vi "process_display.vi"(6 "error in (no error)":errorcluster) -> (0 "error out":errorcluster)   [LabVIEW 2010]
uses:
  typedefs/control_display_enum.ctl
  typedefs/data_array.ctl
panel:
  out "Waveform Chart":waveform(dbl)[](graph)
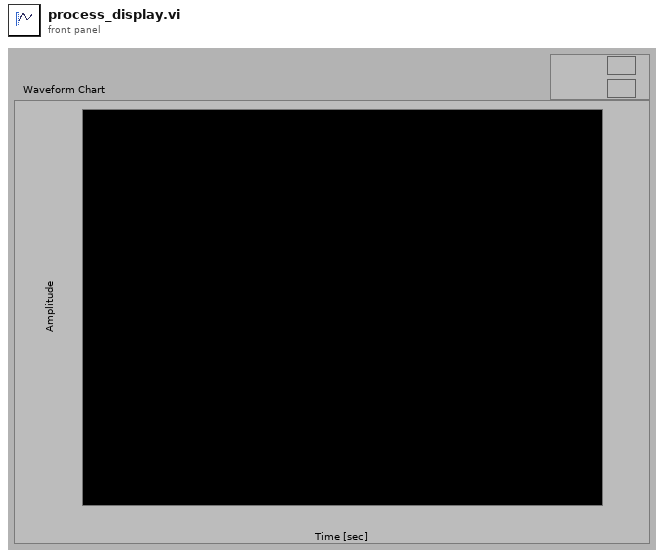
[diagram p1: front panel]
types:
  T1 = typedef "data_array.ctl" = waveform(dbl)[]
  T2 = typedef "control_display_enum.ctl" = enum16{"Init", "Display", "Quit"}
  T3 = cluster{"Control display enum":T2, "variant":variant}
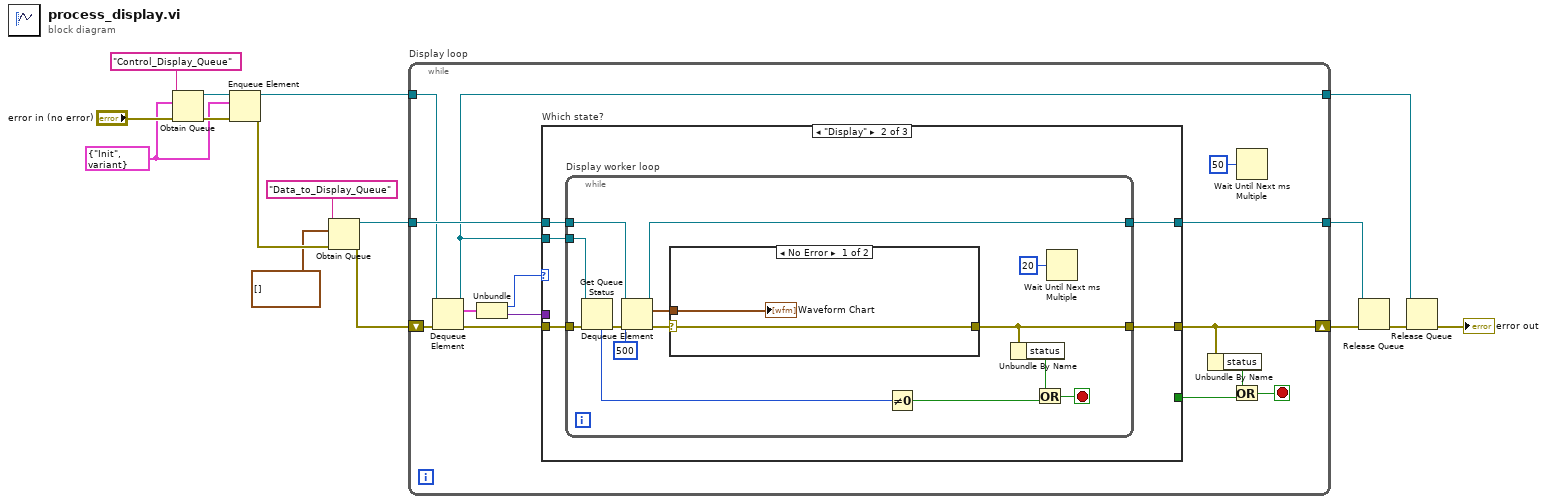
[diagram p0: block diagram]
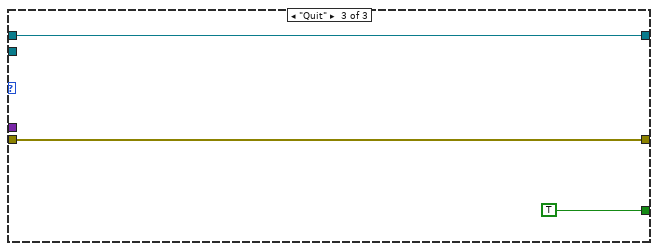
[diagram p4: hidden frame]
diagram:
  w8 = T3 {"Control display enum"=enum."Init", "variant"=variant}
  n1 = Obtain Queue(name (unnamed)="Control_Display_Queue", element data type=w8, error in (no error)="error in (no error)") -> (queue out=w7:refnum<queue>, error out=w10:errorcluster)  [unwired: 2 in, 1 out]
  n2 = Enqueue Element(queue=w7, element=w8, error in (no error)=w10) -> (queue out=w6:refnum<queue>, error out=w9:errorcluster)  [unwired: 1 in, 1 out]
  n3 = Obtain Queue(name (unnamed)="Data_to_Display_Queue", element data type=T1 [] ("Data cluster"), error in (no error)=w9) -> (queue out=w15:refnum<queue>, error out=w16:errorcluster)  [unwired: 2 in, 1 out]
  n4 = while "Display loop" {
    tunnel: w15 -> [w30]
    shift-right: [w29] -> w13
    shift-left: w16 -> [w28]
    tunnel: w6 -> [w26]
    tunnel: [w18] -> w2
    tunnel: [w22] -> w5
    stop <- w19 stop-if-true
    n5 = Dequeue Element(queue=w26, error in (no error)=w28) -> (queue out=w18:refnum<queue>, element=w25:T3, error out=w27:errorcluster)  [unwired: 1 in, 1 out]
    n6 = Unbundle(w25) -> ("Control display enum"=w24:T2, "variant"=w23:variant)
    n7 = case "Which state?" shown="\"Display\"" w24 {
      tunnel: w30 -> [w32 w37 w57]
      tunnel: w27 -> [w31 w36 w55]
      tunnel: [w31 w35 w55] -> w29
      tunnel: w23 -> [_ _ _]
      tunnel: [w32 w34 w57] -> w22
      tunnel: [_ _ TRUE] -> w21
      tunnel: w18 -> [_ w33 _]
      frame "Init", Default {
      }
      frame "Display" {
        n8 = while "Display worker loop" {
          tunnel: w37 -> [w51]
          tunnel: w36 -> [w43]
          tunnel: [w47] -> w35
          tunnel: [w49] -> w34
          tunnel: w33 -> [w39]
          stop <- w45 stop-if-true
          n9 = Get Queue Status(queue=w39, error in (no error)=w43) -> (error out=w42:errorcluster, # elements in queue=w48:i32)  [unwired: 1 in, 6 out]
          n10 = Dequeue Element(queue=w51, timeout in ms (-1)=500, error in (no error)=w42) -> (queue out=w49:refnum<queue>, element=w50:T1, error out=w41:errorcluster)  [unwired: 1 out]
          n11 = case shown="No Error" w41 {
            selector: w41 -> [w53 w54]
            tunnel: [w53 w54] -> w47
            tunnel: w50 -> [w52 _]
            frame No Error {
              "Waveform Chart" <- w52
            }
            frame Error {
            }
          }
          n12 = Not Equal To 0?(x=w48) -> (x != 0?=w44:bool)
          n13 = Unbundle By Name(w47) -> ("status"=w46:bool)
          n14 = Or(x=w46, y=w44) -> (x .or. y?=w45:bool)
          n15 = Wait Until Next ms Multiple(millisecond multiple=u32 20) -> ()  [unwired: 1 out]
        }
      }
      frame "Quit" {
      }
    }
    n16 = Unbundle By Name(w29) -> ("status"=w20:bool)
    n17 = Or(x=w20, y=w21) -> (x .or. y?=w19:bool)
    n18 = Wait Until Next ms Multiple(millisecond multiple=u32 50) -> ()  [unwired: 1 out]
  }
  n19 = Release Queue(queue=w5, error in (no error)=w13) -> (error out=w4:errorcluster)  [unwired: 1 in, 2 out]
  n20 = Release Queue(queue=w2, error in (no error)=w4) -> (error out=→"error out":errorcluster)  [unwired: 1 in, 2 out]
